vi "Write ActorConfiguration.vi"(10 "ActorConfiguration":T1={"GlobalConfiguration"={"DeviceFamily"="", "WriteData"=FALSE, "BufferSize_samples"=-1, "SyncDevice"=FALSE, "ExecuteInterruptRoutine"=FALSE, "InterruptRoutineTimeout_ms"=-1}, "DeviceConfiguration"={"DeviceSpecificName"="MIPI_Camera", "HardwareReference"="PXIe-Slot2", "UsedResources"=[{"ResourceLocation"="FrontFacing", "ResourceData"=variant(string "Use this Variant to store your specific resource data.\nThis will be read from and written to with the JSON parsing API.\nIn the child implementation you can use the acessors provided to convert from the specific cluster to your own device's implementation")}]}}, 11 "Template in":refnum<class "Template.lvclass">) -> (3 "Template out":refnum<class "Template.lvclass">)   [LabVIEW 2020, in "Template.lvlib" / "Template.lvclass"]
doc: "Sets the configuration cluster read from the JSON file\nUpdates the Actors to Nest array using a copy of the base class and the configurations provided in the ActorConfiguration cluster"
uses:
  Template.lvclass
  C:/Program Files/National Instruments/LabVIEW 2020/vi.lib/ActorFramework/Actor/Actor.lvclass
  typedefs/actor configuration.ctl
  typedefs/shared actor configuration.ctl
  typedefs/resource config/device configuration cluster.ctl
  typedefs/resource config/single resource cluster.ctl
  Template.lvclass/Template.ctl
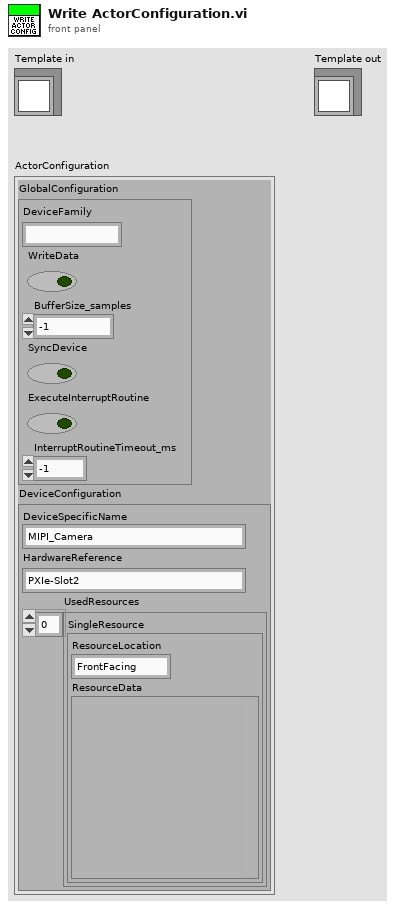
[diagram p1: front panel]
types:
  T1 = typedef "Template.lvlib/Template.lvclass/actor configuration.ctl" = cluster{"GlobalConfiguration":T2, "DeviceConfiguration":T3}
  T2 = typedef "Template.lvlib/Template.lvclass/shared actor configuration.ctl" = cluster{"DeviceFamily":string, "WriteData":bool, "BufferSize_samples":i32, "SyncDevice":bool, "ExecuteInterruptRoutine":bool, "InterruptRoutineTimeout_ms":i32}
  T3 = typedef "Template.lvlib/Template.lvclass/device configuration cluster.ctl" = cluster{"DeviceSpecificName":string, "HardwareReference":string, "UsedResources":T4[]}
  T4 = typedef "Template.lvlib/Template.lvclass/single resource cluster.ctl" = cluster{"ResourceLocation":string, "ResourceData":variant}
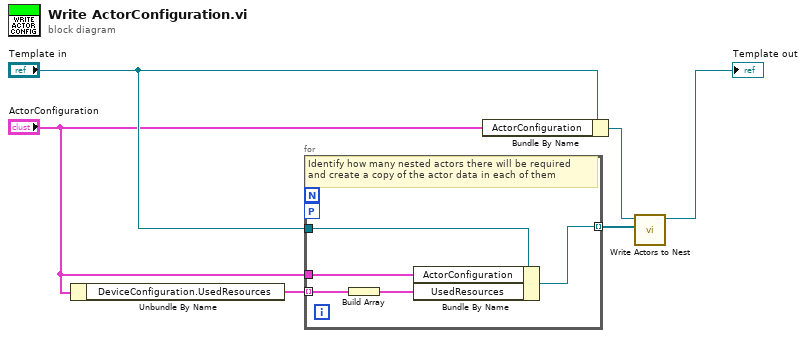
[diagram p0: block diagram]
diagram:
  n1 = Unbundle By Name("ActorConfiguration") -> ("DeviceConfiguration.UsedResources"=w3:T4[])
  n2 = for {
    tunnel: "Template in" -> [w11]
    tunnel: "ActorConfiguration" -> [w9]
    tunnel: [w10] -> w1 mode=indexing
    tunnel: w3 -> [w8] mode=indexing
    workers-P: _ -> [_]
    # "Identify how many nested actors there will be required\nand create a copy of the actor data in each of them"
    n3 = Build Array(w8) -> (w7:T4[])
    n4 = Bundle By Name(cluster=w11, "ActorConfiguration"=w9, "UsedResources"=w7) -> (w10:refnum<class "Template.lvclass">)
  }
  n5 = Bundle By Name(cluster="Template in", "ActorConfiguration"="ActorConfiguration") -> (w6:refnum<class "Template.lvclass">)
  n6 = call "Write Actors to Nest.vi"("Actors to Nest"=w1, "Template in"=w6) -> ("Template out"=→"Template out":refnum<class "Template.lvclass">)  [unwired: 9 in]
